vi "cmd打开文件夹.vi"(7 "模式(打开目录)":enum16{"选择文件", "仅打开目录"}(ring)=enum."仅打开目录", 8 "error in (no error)":errorcluster caption="错误输入（无错误）", 11 "文件路径":path) -> (0 "error out":errorcluster caption="错误输出")   [LabVIEW 2017]
panel:
  out "error out 2":errorcluster caption="错误输出"
  out "selected path":path caption="所选路径"
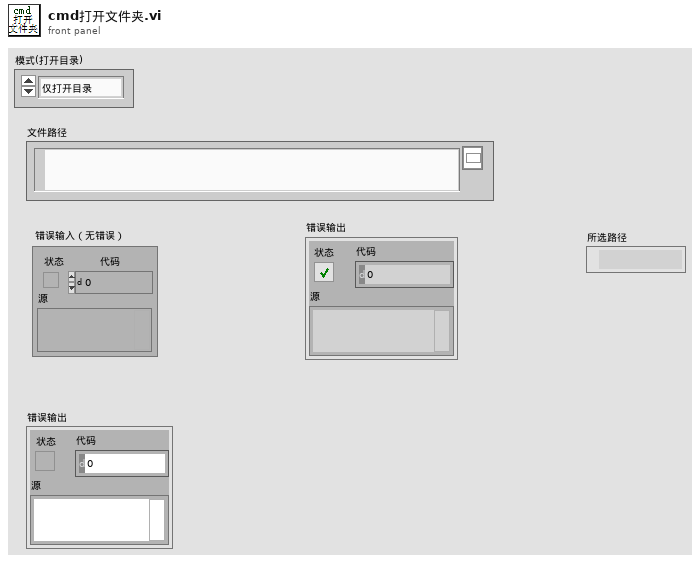
[diagram p1: front panel]
types:
  T1 = enum16{"open", "replace", "create", "open or create", "replace or create", "replace or create with confirmation"}
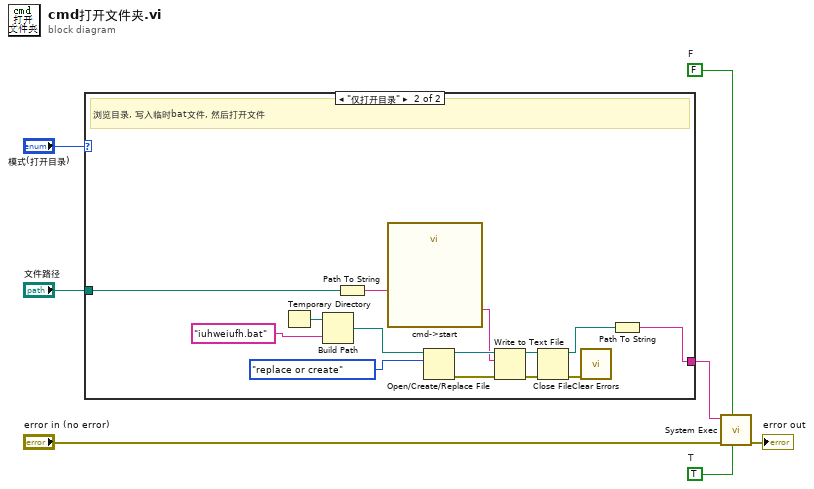
[diagram p0: block diagram]
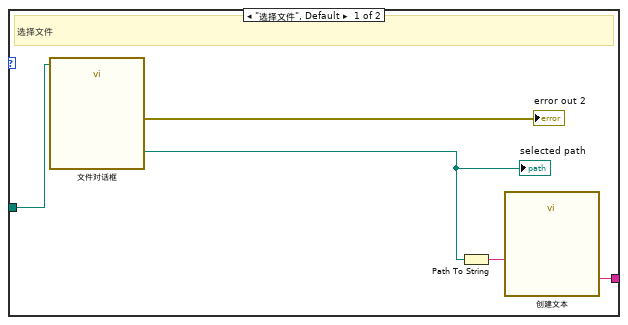
[diagram p2: hidden frame]
diagram:
  w5 = FALSE  # F
  w6 = TRUE  # T
  n1 = case shown="\"仅打开目录\"" "模式(打开目录)" {
    tunnel: "文件路径" -> [w12 w24]
    tunnel: [w11 w16] -> w3
    frame "选择文件", Default {
      # "选择文件"
      n2 = call "文件对话框"("start path"=w12) -> ("selected path"=w8:path, "error out"=→"error out 2":errorcluster)  [unwired: 11 in, 2 out]
      "selected path" <- w8
      n3 = Path To String(path=w8) -> (string=w10:string)
      n4 = call "创建文本"("文件路径"=w10) -> ("Result"=w11:string)  [unwired: 13 in, 1 out]
    }
    frame "仅打开目录" {
      # "浏览目录, 写入临时bat文件, 然后打开文件"
      n5 = Temporary Directory() -> (w26:path)
      n6 = Build Path(base path=w26, name or relative path="iuhweiufh.bat" ("名称或相对路径")) -> (appended path=w22:path)
      n7 = Path To String(path=w24) -> (string=w14:string)
      n8 = call "cmd->start"("路径"=w14) -> ("Result"=w13:string)  [unwired: 13 in, 1 out]
      n9 = Open/Create/Replace File(file path (use dialog)=w22, operation (0:open)=T1."replace or create" ("操作(0:open)")) -> (refnum out=w21:refnum<file>, error out=w19:errorcluster)  [unwired: 4 in, 1 out]
      n10 = Write to Text File(file (use dialog)=w21, text=w13, error in=w19) -> (refnum out=w20:refnum<file>, error out=w18:errorcluster)  [unwired: 1 in, 1 out]
      n11 = Close File(refnum=w20, error in=w18) -> (path=w17:path, error out=w15:errorcluster)
      n12 = call <vilib>:"Clear Errors.vi"("error in (no error)"=w15) -> ()  [unwired: 5 in, 2 out]
      n13 = Path To String(path=w17) -> (string=w16:string)
    }
  }
  n14 = call <vilib>:"System Exec.vi"("run minimized? (F)"=w6, "wait until completion? (T)"=w5, "error in (no error)"="error in (no error)", "command line"=w3) -> ("error out"=→"error out":errorcluster)  [unwired: 4 in, 3 out]
